vi "ActorDatabase-Initialize.vi"(8 "error in (no error)":errorcluster, 11 "Database-Actor In":refnum<class "PartCertDatabase-Actor.lvclass">) -> (0 "error out":errorcluster, 3 "Database-Actor out":refnum<class "PartCertDatabase-Actor.lvclass">)   [LabVIEW 2013, in "PartCertDatabase-Actor.lvclass"]
uses:
  PartCertDatabase-Actor.lvclass
  PartCertDatabase-Actor.lvclass/PartCertDatabase-Actor.ctl
  Reuse Library/Database API/PartCertDatabase-API.lvclass
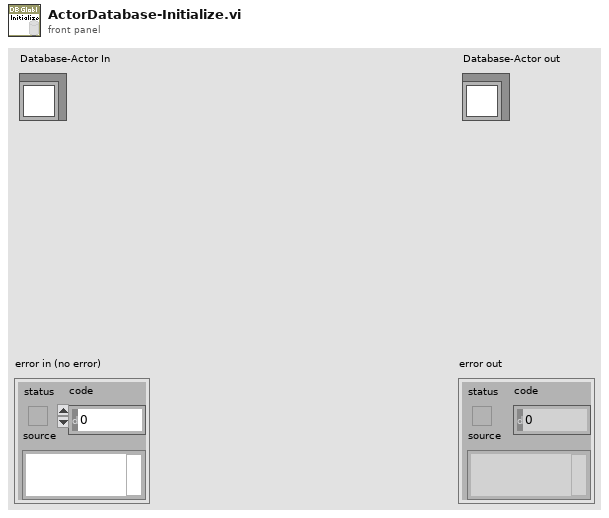
[diagram p1: front panel]
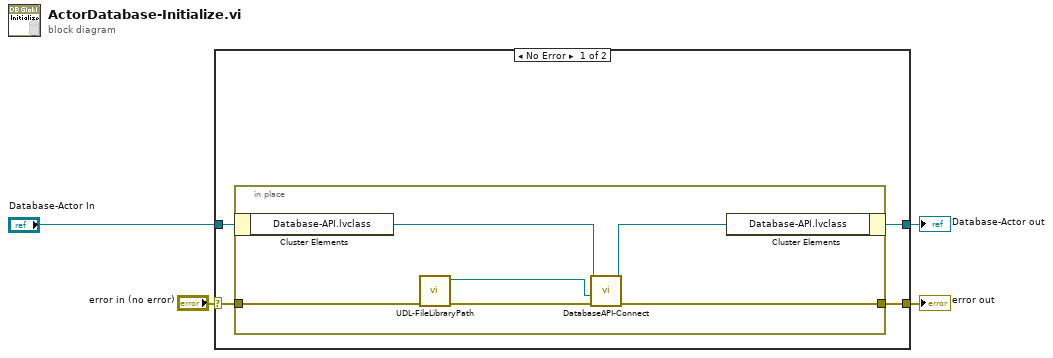
[diagram p0: block diagram]
diagram:
  n1 = case shown="No Error" "error in (no error)" {
    selector: "error in (no error)" -> [w7 w16]
    tunnel: [w6 w16] -> w3
    tunnel: [w8 w15] -> w2
    tunnel: "Database-Actor In" -> [w5 w15]
    frame No Error {
      n2 = in-place {
        in-place-border: w7 -> [w11]
        in-place-border: [w12] -> w6
        n3 = in-place-cluster #1(w5) -> ("Database-API.lvclass"=w14:refnum<class "PartCertDatabase-API.lvclass">)
        n4 = call "UDL-FileLibraryPath.vi"("error in"=w11) -> ("error out"=w10:errorcluster, "Library Filepath"=w9:path)  [unwired: 9 in]
        n5 = call "DatabaseAPI-Connect.vi"("error in (no error)"=w10, "Database (mdb)  File Path"=w9, "Database-API in"=w14) -> ("error out"=w12:errorcluster, "Database-API out"=w13:refnum<class "PartCertDatabase-API.lvclass">)  [unwired: 7 in]
        n6 = in-place-cluster #1("Database-API.lvclass"=w13) -> (w8:refnum<class "PartCertDatabase-Actor.lvclass">)
      }
    }
    frame Error {
    }
  }
  "error out" <- w3
  "Database-Actor out" <- w2
